vi "QSM_CreateRef.vi"(8 "error in":errorcluster) -> (0 "error out":errorcluster, 3 "Test QSM_Reference out":T1)   [LabVIEW 2014, in "TestQSM.lvlib"]
doc: "VARIABLE FREQUENCY DRIVE CONTROL 'VFDC' Queued State Machine Shift Register Data:\n\nThe data type for the main shift register in the subsequent queued state machine is defined in large clusters within this VI."
uses:
  Controls/QSM_Reference.ctl
  Controls/QSM_DataType.ctl
  Controls/QSM_RunStates.ctl
  TestQSM.lvlib
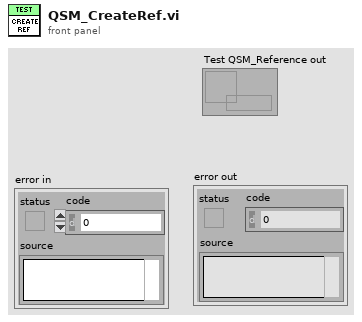
[diagram p1: front panel]
types:
  T1 = typedef "TestQSM.lvlib/QSM_Reference.ctl" = refnum<queue>
  T2 = typedef "TestQSM.lvlib/QSM_DataType.ctl" = cluster{"RunStates":T3, "Data (Variant)":variant}
  T3 = typedef "TestQSM.lvlib/QSM_RunStates.ctl" = enum16{"NULL", "Sect01-Initialize-00-GROUP.ENQUEUE", "Sect02-Single File_Check for Parameters", "Sect02-Single File_Ask for File", "Sect02-Single File_Run Analysis", "Sect02-Single File_Write Results", "Sect03-Single ROI Calc_Check for Parameters", "Sect03-Single ROI Calc_Ask for File", "Sect03-Single ROI Calc_Run Analysis", "Sect03-Single ROI _Write Results", "Sect12-Full Dir_Check for Parameters", "Sect12-Full Dir_Ask for Dir", "Sect12-Full Dir_Check for Next Image to Process", "Sect12-Full Dir_Run Analysis", "Sect12-Full Dir_Write Results", "Sect12-Full Dir_Check if User Stopped", "Sect13-FullDir ROI Calc_Check for Parameters", "Sect13-FullDir ROI Calc_Ask for Dir", "Sect13-Full Dir ROI Calc_Check for Next Image to Process", "Sect13-Full Dir ROI Calc_Run Analysis", "Sect13-Full Dir ROI Calc_Write Results", "Sect13-Full Dir ROI Calc_Check if User Stopped", "Sect90-GUI_Config_Change UI Before Analysis", "Sect90-GUI_Config_Change UI After Analysis", "Sect90-GUI_Stop Processing Pressed", "Sect90-GUI_Stop Processing Button Set Back to F", "Sect90-GUI_Clear ROIs", "Sect99_EXIT-00-Group.Enqueue", "Sect99_EXIT-01-StopQSM"}
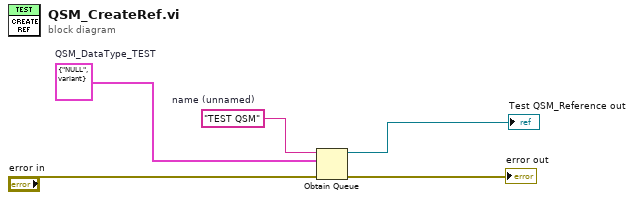
[diagram p0: block diagram]
diagram:
  w5 = T2 {"RunStates"=enum."NULL", "Data (Variant)"=variant}  # QSM_DataType_TEST
  w2 = "TEST QSM"  # name (unnamed)
  n1 = Obtain Queue ("Obtain Queues")(name (unnamed)=w2, element data type=w5, error in (no error)="error in") -> (queue out=→"Test QSM_Reference out":refnum<queue>, error out=→"error out":errorcluster)  [unwired: 2 in, 1 out]
